vi "get_time.vi"(1 "input cluster":T3) -> (0 "millisecond timer value":u32)   [LabVIEW 2015]
uses:
  <vilib>/vision/Avi1.llb/AviRefnum.ctl
  <vilib>/userdefined/High Color/IMAQdx.ctl
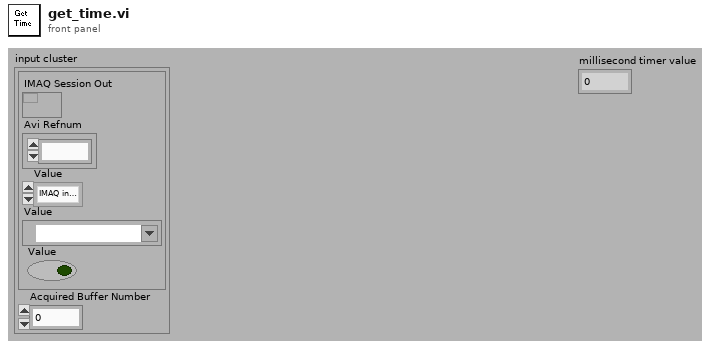
[diagram p1: front panel]
types:
  T1 = typedef "AviRefnum.ctl" = refnum<k1>
  T2 = typedef "IMAQdx.ctl" = refnum<k21>
  T3 = cluster{cluster{"IMAQ Session Out":refnum<k11>, "Avi Refnum":T1, "Value":enum32{"IMAQ interface", "IMAQdx interface", "AVI file"}, "Value":T2, "Value":bool}, "Acquired Buffer Number":i32}
  T4 = cluster{"IMAQ Session Out":refnum<k11>, "Avi Refnum":T1, "Value":enum32{"IMAQ interface", "IMAQdx interface", "AVI file"}, "Value":T2, "Value":bool}
  T5 = enum32{"IMAQ interface", "IMAQdx interface", "AVI file"}
  T6 = cluster{"width":u32, "height":u32, "framesPerSecond":u32, "compressionFilter":string, "hasData":bool}
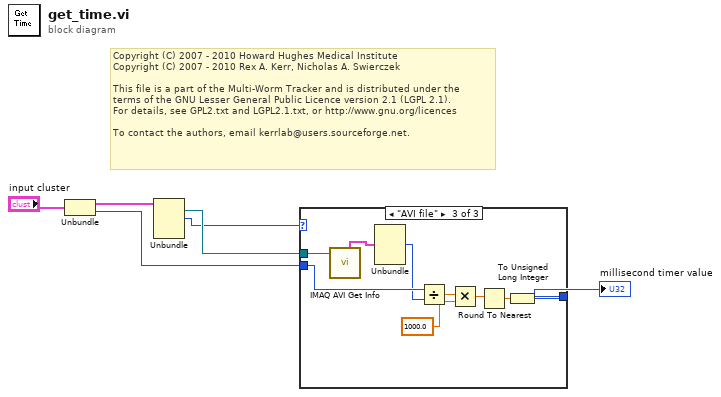
[diagram p0: block diagram]
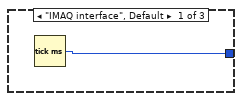
[diagram p2: hidden frame]
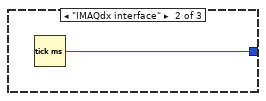
[diagram p3: hidden frame]
diagram:
  # "Copyright (C) 2007 - 2010 Howard Hughes Medical Institute\nCopyright (C) 2007 - 2010 Rex A. Kerr, Nicholas A. Swierczek\n \nThis file is a part of the Multi-Worm Tracker and is distributed under the\nterms of the GNU Lesser General Public Licence version 2.1 (LGPL 2.1).\nFor details, see GPL2.txt and LGPL2.1.txt, or http://www.gnu.org/licences\n \nTo contact the authors, email kerrlab@users.sourceforge.net."
  n1 = Unbundle("input cluster") -> (w6:T4, "Acquired Buffer Number"=w5:i32)
  n2 = Unbundle(w6) -> ("Avi Refnum"=w3:T1, "Value"=w2:T5)  [unwired: 3 out]
  n3 = case shown="\"AVI file\"" w2 {
    tunnel: [w7 w8 w12] -> w4
    tunnel: w5 -> [_ _ w15]
    tunnel: w3 -> [_ _ w17]
    frame "IMAQ interface", Default {
      n4 = Tick Count (ms)() -> (millisecond timer value=w7:u32)
    }
    frame "IMAQdx interface" {
      n5 = Tick Count (ms)() -> (millisecond timer value=w8:u32)
    }
    frame "AVI file" {
      n6 = call "IMAQ AVI Get Info"("Avi Refnum"=w17) -> ("Frame Data"=w16:T6)  [unwired: 6 in, 4 out]
      n7 = Unbundle(w16) -> ("framesPerSecond"=w14:u32)  [unwired: 4 out]
      n8 = Divide(x=w15, y=w14) -> (x/y=w11:dbl)
      n9 = Multiply(x=w11, y=1000.0) -> (x*y=w9:dbl)
      n10 = Round To Nearest(number=w9) -> (nearest integer value=w13:dbl)
      n11 = To Unsigned Long Integer(number=w13) -> (unsigned 32bit integer=w12:u32)
    }
  }
  "millisecond timer value" <- w4
